vi "Stop Nested Models.vi"(8 "error in (no error)":errorcluster, 11 "IModel in":refnum<class "IModel.lvclass">) -> (0 "error out":errorcluster, 2 "Tracked Actors Running":i32, 3 "IModel out":refnum<class "IModel.lvclass">)   [LabVIEW 2017, in "IModel.lvlib" / "IModel.lvclass"]
uses:
  <vilib>/gpm_packages/@cs/mva-core/Source/IModel/IModel/IModel.lvclass
  <vilib>/gpm_packages/@cs/mva-core/Source/IModel/IModel/IModel.lvclass/IModel.ctl
  <vilib>/ActorFramework/Message Enqueuer/Message Enqueuer.lvclass
  <vilib>/ActorFramework/Message Enqueuer/Message Enqueuer.lvclass/Message Enqueuer.ctl
  <vilib>/ActorFramework/Message Enqueuer/Enqueue.vi
  <vilib>/ActorFramework/Stop Msg/Stop Msg.lvclass
  C:/Program Files/National Instruments/LabVIEW 2017/vi.lib/ActorFramework/Message/Message.lvclass
  <vilib>/ActorFramework/Message Priority Queue/Priority Enqueue.vi
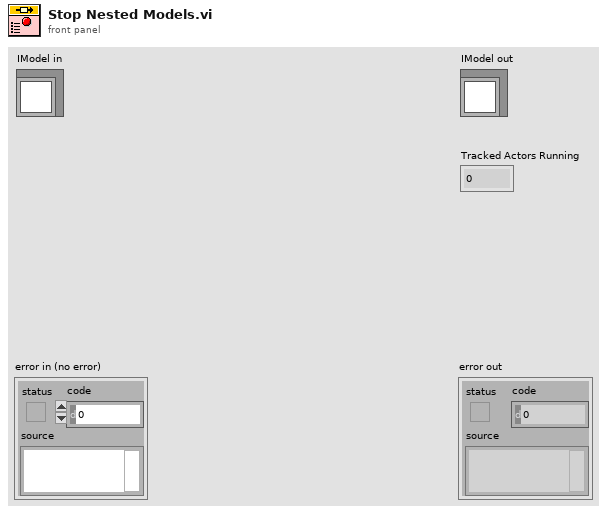
[diagram p1: front panel]
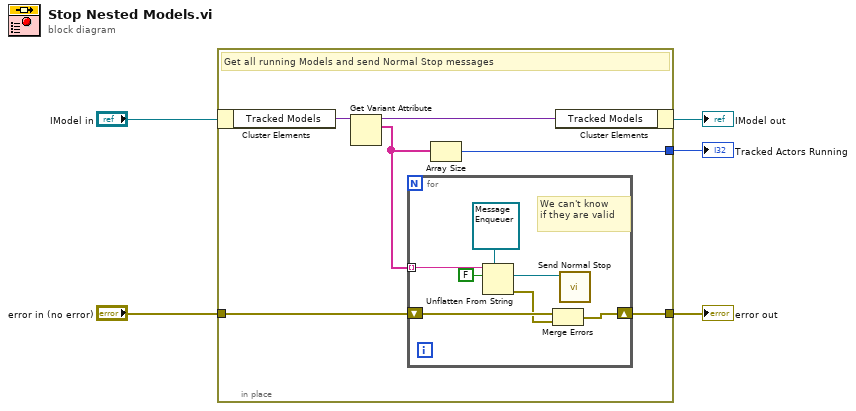
[diagram p0: block diagram]
diagram:
  n1 = in-place {
    in-place-border: "error in (no error)" -> [w9]
    in-place-border: [w8] -> w2
    in-place-border: [w6] -> w1
    # "Get all running Models and send Normal Stop messages"
    n2 = in-place-cluster #1("IModel in") -> ("Tracked Models"=w11:variant)
    n3 = Get Variant Attribute(Variant=w11) -> (duplicate Variant=w10:variant, names=w7:string[])  [unwired: 3 in, 2 out]
    n4 = for {
      tunnel: w7 -> [w18] mode=indexing
      shift-right: [w16] -> w8
      shift-left: w9 -> [w15]
      # "We can't know\nif they are valid"
      n5 = Unflatten From String(type=refnum<class "Message Enqueuer.lvclass"> refnum ("Nested Model Enqueuer"), binary string=w18, data includes array or string size? (T)=FALSE) -> (value=w13:refnum<class "Message Enqueuer.lvclass">, error out=w14:errorcluster)  [unwired: 2 in, 1 out]
      n6 = Merge Errors(w15, w14) -> (w16:errorcluster)
      n7 = call <vilib>:"Send Normal Stop.vi"("Message Enqueuer"=w13) -> ()  [unwired: 10 in, 1 out]
    }
    n8 = Array Size(array=w7) -> (size(s)=w6:i32)
    n9 = in-place-cluster #1("Tracked Models"=w10) -> (→"IModel out":refnum<class "IModel.lvclass">)
  }
  "error out" <- w2
  "Tracked Actors Running" <- w1
